vi "Get Menu Pane Reference.vi"(8 "error in (no error)":errorcluster, 11 "SwipeMenu in":refnum<class "SwipeMenu.lvclass">) -> (0 "error out":errorcluster, 2 "Menu Pane Refnum":refnum<vi>, 3 "SwipeMenu out":refnum<class "SwipeMenu.lvclass">)   [LabVIEW 2019, in "SwipeMenu.lvclass"]
uses:
  SwipeMenu.lvclass
  C:/Program Files (x86)/National Instruments/LabVIEW 2019/vi.lib/QSI/QControls/QControl Classes/SubPanel/SubPanel.lvclass
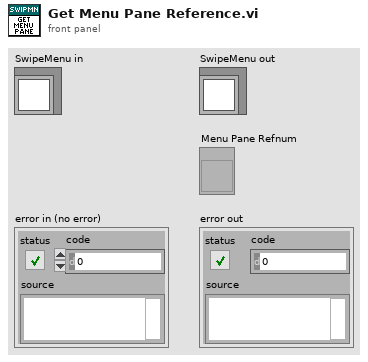
[diagram p1: front panel]
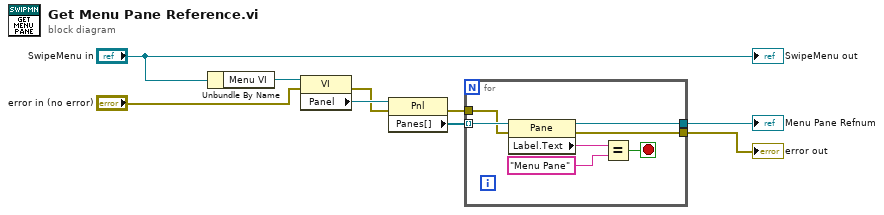
[diagram p0: block diagram]
diagram:
  n1 = Unbundle By Name("SwipeMenu in") -> ("Menu VI"=w3:refnum<vi>)
  n2 = property class="VI"(reference=w3, error in="error in (no error)") -> (error out=w8:errorcluster, "Panel"=w9:refnum<vi>)  [unwired: 1 out]
  n3 = property class="Pnl"(reference=w9, error in=w8) -> (error out=w6:errorcluster, "Panes[]"=w7:refnum<vi>[])  [unwired: 1 out]
  n4 = for {
    tunnel: w7 -> [w16] mode=indexing
    tunnel: w6 -> [w14]
    tunnel: [w11] -> w5
    tunnel: [w10] -> w4
    stop <- w13 stop-if-true
    n5 = property class="Pane"(reference=w16, error in=w14) -> (reference out=w11:refnum<vi>, error out=w10:errorcluster, "Label.Text"=w15:string)
    n6 = Equal?(x=w15, y="Menu Pane") -> (x = y?=w13:bool)
  }
  "Menu Pane Refnum" <- w5
  "error out" <- w4
  "SwipeMenu out" <- "SwipeMenu in"
